vi "Set Timeouts.vi"(8 "error in (no error)":errorcluster, 9 "write operation timeout (ms)":i32=5000, 10 "read operation timeout (ms)":i32=5000, 11 "Modbus master in":refnum<class "Modbus Master.lvclass">) -> (0 "error out":errorcluster, 3 "Modbus master out":refnum<class "Modbus Master.lvclass">)   [LabVIEW 2015, in "Modbus Master.lvclass"]
doc: "Sets both read and write operation timeouts on a Modbus slave."
uses:
  <vilib>/Modbus/master/Modbus Master.lvclass
  <vilib>/Modbus/subvis/Modbus API/Modbus API.lvclass/Modbus API.ctl
  <vilib>/Modbus/subvis/Transmission Data Unit (ADU)/Transmission Data Unit/Transmission Data Unit.lvclass/Transmission Data Unit.ctl
  <vilib>/Modbus/subvis/Transmission Data Unit (ADU)/Transmission Data Unit/Transmission Data Unit.lvclass
  <vilib>/Modbus/subvis/Modbus API/Modbus API.lvclass
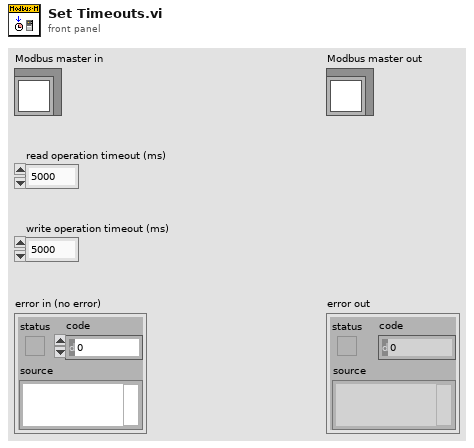
[diagram p1: front panel]
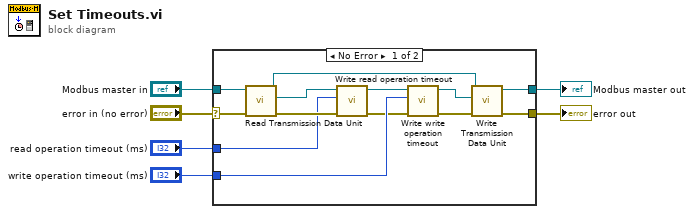
[diagram p0: block diagram]
diagram:
  n1 = case shown="No Error" "error in (no error)" {
    selector: "error in (no error)" -> [w7 w21]
    tunnel: "write operation timeout (ms)" -> [w14 _]
    tunnel: "read operation timeout (ms)" -> [w13 _]
    tunnel: [w10 w20] -> w4
    tunnel: [w9 w21] -> w3
    tunnel: "Modbus master in" -> [w8 w20]
    frame No Error {
      n2 = call <vilib>:"Read Transmission Data Unit.vi"("error in (no error)"=w7, "Modbus instance in"=w8) -> ("error out"=w17:errorcluster, "transmission data unit"=w18:refnum<class "Transmission Data Unit.lvclass">, "Modbus instance out"=w19:refnum<class "Modbus Master.lvclass">)  [unwired: 7 in]
      n3 = call <vilib>:"Write read operation timeout.vi"("error in (no error)"=w17, "read operation timeout"=w13, "transmission data unit in"=w18) -> ("error out"=w12:errorcluster, "transmission data unit out"=w15:refnum<class "Transmission Data Unit.lvclass">)  [unwired: 7 in]
      n4 = call <vilib>:"Write write operation timeout.vi"("error in (no error)"=w12, "write operation timeout"=w14, "transmission data unit in"=w15) -> ("error out"=w11:errorcluster, "transmission data unit out"=w16:refnum<class "Transmission Data Unit.lvclass">)  [unwired: 7 in]
      n5 = call <vilib>:"Write Transmission Data Unit.vi"("error in (no error)"=w11, "transmission data unit"=w16, "Modbus instance in"=w19) -> ("error out"=w9:errorcluster, "Modbus instance out"=w10:refnum<class "Modbus Master.lvclass">)  [unwired: 7 in]
    }
    frame Error {
    }
  }
  "error out" <- w3
  "Modbus master out" <- w4
